vi "Buff TimeStamp Into Que.vi"(10 "Logging Cluster":T1 {"Exp params"."TSFrames" min=1 step=1; "Exp params"."TSfps" min=0.001 max=90.0 step=0.001 format="%_4g"}, 11 "Queue in":refnum<queue>) -> (2 "Logging Cluster out":T1 {"Exp params"."TSFrames" min=1 step=1; "Exp params"."TSfps" min=0.001 max=90.0 step=0.001 format="%_4g"})   [LabVIEW 2020]
uses:
  _controls/Logging Cluster.ctl
  _controls/Exp Params.ctl
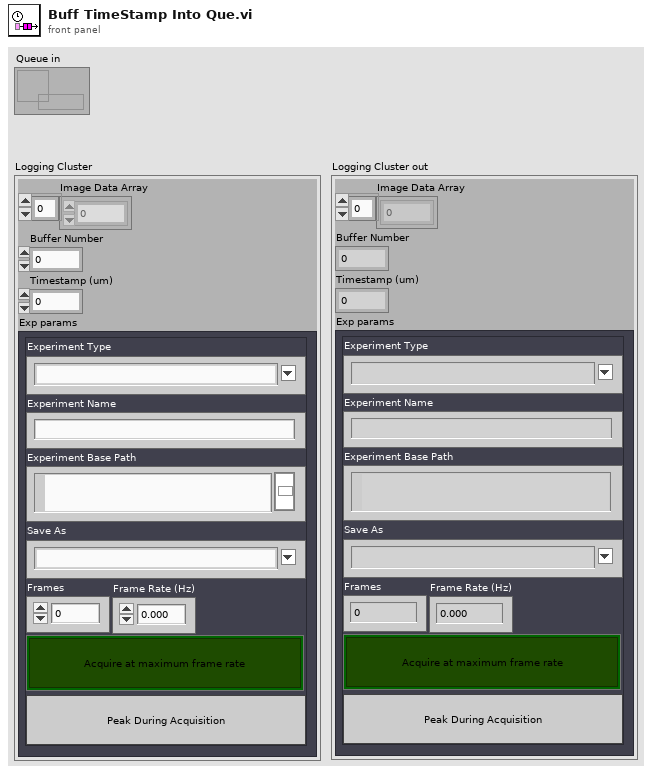
[diagram p1: front panel]
types:
  T1 = typedef "Logging Cluster.ctl" = cluster{"Image Data Array":u8[], "Buffer Number":i32, "Timestamp (um)":u64, "Exp params":T2}
  T2 = typedef "Exp Params.ctl" = cluster{"Experiment Type":string, "Experiment Name":string, "ExpPath":path, "Save As":string, "TSFrames":i32, "TSfps":dbl, "Streaming":bool, "tdms ref":refnum<k34>, "frame #":i64, "Full Path":path, "PeakOnQueue":bool}
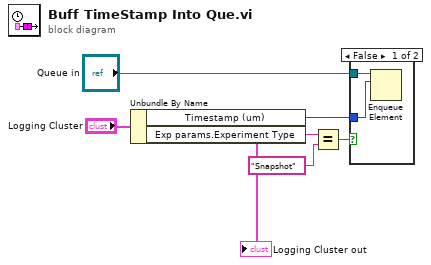
[diagram p0: block diagram]
diagram:
  n1 = Unbundle By Name("Logging Cluster") -> ("Timestamp (um)"=w6:u64, "Exp params.Experiment Type"=w4:string)
  n2 = Equal?(x=w4, y="Snapshot") -> (x = y?=w1:bool)
  n3 = case shown="False" w1 {
    tunnel: "Queue in" -> [w8 _]
    tunnel: w6 -> [w7 _]
    frame False {
      n4 = Enqueue Element(queue=w8, element=w7) -> ()  [unwired: 2 in, 3 out]
    }
    frame True {
    }
  }
  "Logging Cluster out" <- "Logging Cluster"
